vi "Communication VISA mMc.vi"(0 "Clr buffer":bool, 1 "Port":T1={"P type"=0, "reference"="", " Terminator "="\r\n", "Timeout"=300} {"Timeout" step=10; "P type" items=["none", "RS-232C"]}, 2 "Command":string, 3 "error in (no error)":errorcluster, 8 "Term. on Ret.?":bool=TRUE) -> (5 "raw ret":string, 6 "Comm log":string, 7 "Return":string, 9 "error out":errorcluster)   [LabVIEW 2021]
panel:
  out "T Rx":string
  out "T Tx":string
  out "timeout":bool
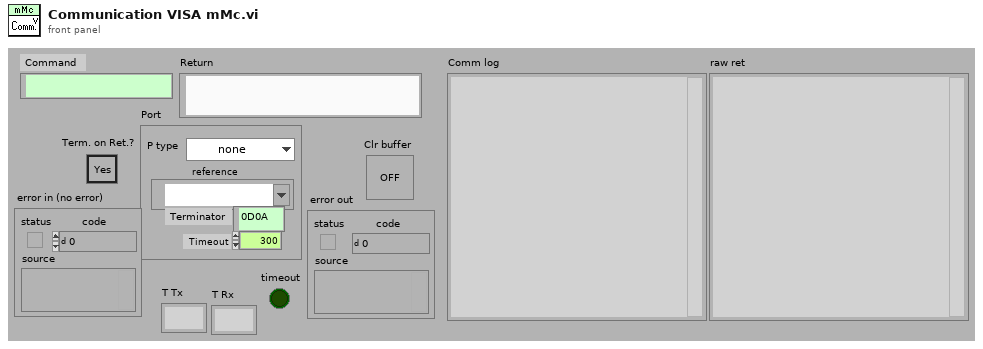
[diagram p1: front panel]
types:
  T1 = cluster{"P type":u16, "reference":refnum<visa-resource-name>, " Terminator ":string, "Timeout":i32}
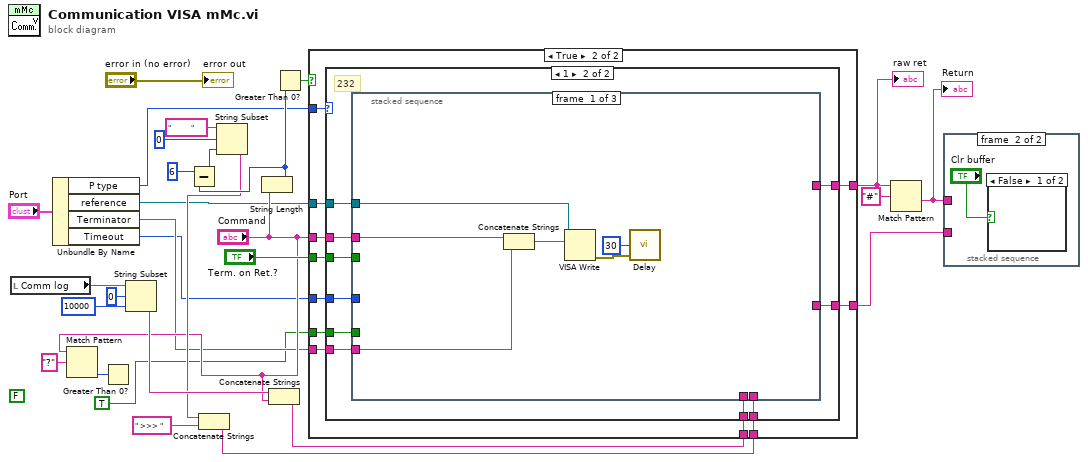
[diagram p0: block diagram]
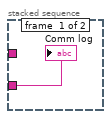
[diagram p2: hidden frame]
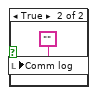
[diagram p3: hidden frame]
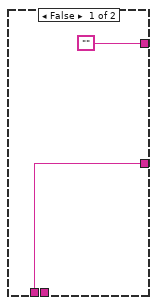
[diagram p4: hidden frame]
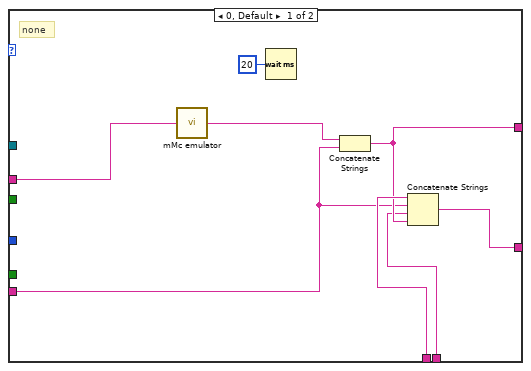
[diagram p5: hidden frame]
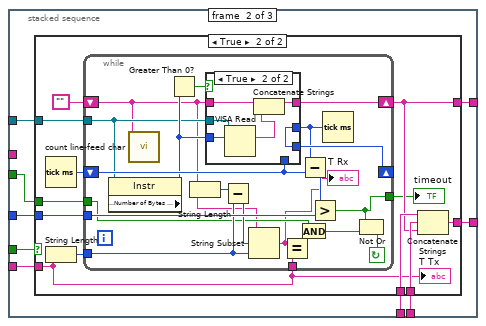
[diagram p6: hidden frame]
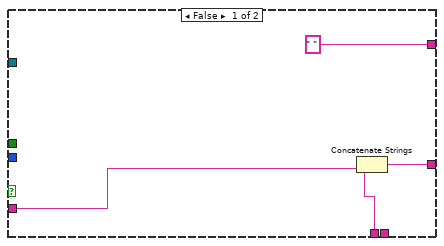
[diagram p7: hidden frame]
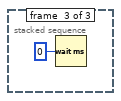
[diagram p9: hidden frame]
diagram:
  (unwired) FALSE
  n1 = local read "Comm log"() -> (w29:string)
  n2 = Unbundle By Name("Port") -> ("P type"=w6:u16, "reference"=w5:refnum<visa-resource-name>, "Terminator"=w4:string, "Timeout"=w3:i32)
  n3 = Match Pattern(string="Command", regular expression="?") -> (offset past match=w8:i32)  [unwired: 1 in, 3 out]
  n4 = Greater Than 0?(x=w8) -> ()  [unwired: 1 out]
  n5 = String Subset(string=w29, offset (0)=0, length (rest)=10000 ("length (rest)")) -> (substring=w23:string)
  n6 = String Length(string="Command") -> (length=w19:i32)
  n7 = Subtract(x=6, y=w19) -> (x-y=w14:i32)
  n8 = String Subset(string="          ", offset (0)=0, length (rest)=w14) -> (substring=w17:string)
  n9 = Concatenate Strings(w17, " >>> " ("Substring")) -> (w15:string)
  n10 = Concatenate Strings(w23, "Command") -> (w21:string)
  n11 = Greater Than 0?(x=w19) -> (x > 0?=w24:bool)
  n12 = case shown="True" w24 {
    tunnel: TRUE -> [_ w42]
    tunnel: w6 -> [_ w41]
    tunnel: w5 -> [_ w40]
    tunnel: ["" w39] -> w1
    tunnel: "Command" -> [_ w38]
    tunnel: w3 -> [_ w37]
    tunnel: "Term. on Ret.?" -> [_ w36]
    tunnel: w4 -> [_ w35]
    tunnel: w21 -> [w30 w34]
    tunnel: [w30 w33] -> w22
    tunnel: w15 -> [_ w32]
    frame False {
    }
    frame True {
      n13 = case shown="1" w41 {
        tunnel: w40 -> [_ w60]
        tunnel: w35 -> [w44 w59]
        tunnel: [w46 w58] -> w39
        tunnel: w38 -> [w50 w57]
        tunnel: w42 -> [_ w56]
        tunnel: w37 -> [_ w55]
        tunnel: w36 -> [_ w54]
        tunnel: w34 -> [w49 w53]
        tunnel: [w48 w52] -> w33
        tunnel: w32 -> [w45 w51]
        frame 0, Default {
          # "none"
          n14 = call "mMc emulator.vi"("Command"=w50) -> ("Return"=w47:string)  [unwired: 7 in, 1 out]
          n15 = Wait (ms)(milliseconds to wait=u32 20) -> ()  [unwired: 1 out]
          n16 = Concatenate Strings(w47, w44) -> (w46:string)
          n17 = Concatenate Strings(w49, w44, w45, w46) -> (w48:string)
        }
        frame 1 {
          # "232"
          n18 = stacked-sequence {
            tunnel: w60 -> [w64 w75 _]
            tunnel: w59 -> [w66 w74 _]
            tunnel: [_ w73 _] -> w58
            tunnel: w57 -> [w65 _ _]
            tunnel: w56 -> [_ w72 _]
            tunnel: w55 -> [_ w71 _]
            tunnel: w54 -> [_ w70 _]
            tunnel: w53 -> [_ w69 _]
            tunnel: [_ w68 _] -> w52
            tunnel: w51 -> [_ w67 _]
            frame #0 {
              n19 = Concatenate Strings(w65, w66) -> (w63:string)
              n20 = VISA Write(VISA resource name=w64, write buffer=w63) -> (error out=w62:errorcluster)  [unwired: 1 in, 2 out]
              n21 = call "Delay.vi"("milliseconds to wait"=u32 30, "error in (no error)"=w62) -> ()  [unwired: 5 in, 3 out]
            }
            frame #1 {
              n22 = case shown="True" w72 {
                tunnel: w71 -> [_ w91]
                tunnel: w75 -> [_ w90]
                tunnel: w74 -> [w77 w80]
                tunnel: [" " ("Substring") w82] -> w73
                tunnel: w70 -> [_ w87]
                tunnel: w69 -> [w78 w85]
                tunnel: [w79 w86] -> w68
                tunnel: w67 -> [_ w84]
                frame False {
                  n23 = Concatenate Strings(w78, w77) -> (w79:string)
                }
                frame True {
                  n24 = Tick Count (ms)() -> (millisecond timer value=w83:u32)
                  n25 = String Length(string=w80) -> (length=w88:i32)
                  n26 = while {
                    tunnel: w87 -> [w100]
                    tunnel: w80 -> [w102]
                    tunnel: w88 -> [w104]
                    shift-left: "" -> [w92]
                    shift-right: [w108] -> w82
                    tunnel: w90 -> [w96]
                    tunnel: w91 -> [w110]
                    shift-left: w83 -> [w105]
                    shift-right: [w107] -> _
                    tunnel: [w95] -> w81
                    stop <- w101 continue-if-true
                    n27 = property class="Instr"(reference=w96) -> ("Serial Settings:Number of Bytes at Serial Port"=w97:u32)  [unwired: 1 in, 2 out]
                    n28 = call "count line-feed char.vi"("string"=w92) -> ()  [unwired: 9 in]
                    n29 = Greater Than 0?(x=w97) -> (x > 0?=w109:bool)
                    n30 = String Length(string=w92) -> (length=w93:i32)
                    n31 = Subtract(x=w93, y=w104) -> (x-y=w103:i32)
                    n32 = String Subset(string=w92, offset (0)=w103, length (rest)=w104) -> (substring=w94:string)
                    "T Rx" <- w94
                    n33 = Equal?(x=w94, y=w102) -> (x = y?=w99:bool)
                    n34 = And(x=w100, y=w99) -> (x .and. y?=w98:bool)
                    n35 = Tick Count (ms)() -> (millisecond timer value=w106:u32)
                    n36 = case shown="True" w109 {
                      tunnel: w96 -> [_ w116]
                      tunnel: w97 -> [_ w115]
                      tunnel: w92 -> [w113 w119]
                      tunnel: [w113 w118] -> w108
                      tunnel: [w112 w117] -> w107
                      tunnel: w106 -> [_ w117]
                      tunnel: w105 -> [w112 _]
                      frame False {
                      }
                      frame True {
                        n37 = VISA Read(VISA resource name=w116, byte count=w115) -> (read buffer=w114:string)  [unwired: 1 in, 3 out]
                        n38 = Concatenate Strings(w119, w114) -> (w118:string)
                      }
                    }
                    n39 = Subtract(x=w106, y=w105) -> (x-y=w111:u32)
                    n40 = Greater?(x=w111, y=w110) -> (0:w95:bool)
                    n41 = Not Or(1:w98, 2:w95) -> (0:w101:bool)
                  }
                  "timeout" <- w81
                  n42 = Concatenate Strings(w85, w84, w82) -> (w86:string)
                  "T Tx" <- w80
                }
              }
            }
            frame #2 {
              n43 = Wait (ms)(milliseconds to wait=u32 0) -> ()  [unwired: 1 out]
            }
          }
        }
      }
    }
  }
  "raw ret" <- w1
  n44 = Match Pattern(string=w1, regular expression="#") -> (after substring=w11:string)  [unwired: 1 in, 3 out]
  "Return" <- w11
  n45 = stacked-sequence {
    tunnel: w11 -> [_ _]
    tunnel: w22 -> [w121 _]
    frame #0 {
      "Comm log" <- w121
    }
    frame #1 {
      n46 = case shown="False" "Clr buffer" {
        frame False {
        }
        frame True {
          n47 = local write "Comm log"("") -> ()
        }
      }
    }
  }
  "error out" <- "error in (no error)"
